vi "calibrationSpectrometer_logEvent_SummaryState.vi"(8 "error in (no error)":errorcluster, 11 "logevent_SummaryState_Ctl":T1) -> (0 "error out":errorcluster, 2 "function return":i32, 3 "logevent_SummaryState_Ctl out":T1)   [LabVIEW 2016, in "SALLV_calibrationSpectrometer.lvlib"]
doc: "int calibrationSpectrometer_shm_logEvent_SummaryStateLV(calibrationSpectrometer_logevent_SummaryStateLV *logevent_SummaryState_Ctl );"
uses:
  SALLV_calibrationSpectrometer.lvlib
  DataTypes/logevent_SummaryState.ctl
  SALLV_calibrationSpectrometer.so
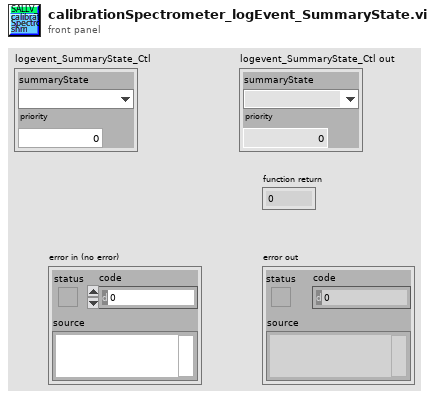
[diagram p1: front panel]
types:
  T1 = typedef "SALLV_calibrationSpectrometer.lvlib/logevent_SummaryState.ctl" = cluster{"summaryState":enum16{"", "DisabledState", "EnabledState", "FaultState", "OfflineState", "StandbyState"}, "priority":i32}
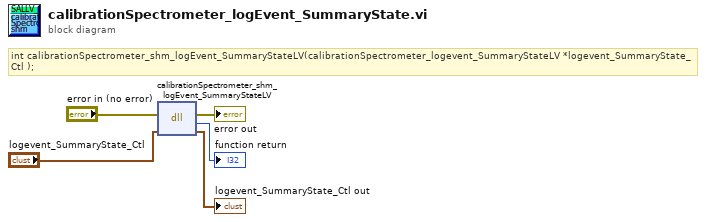
[diagram p0: block diagram]
diagram:
  # "int calibrationSpectrometer_shm_logEvent_SummaryStateLV(calibrationSpectrometer_logevent_SummaryStateLV *logevent_SummaryState_Ctl );"
  n1 = dll-call lib="home/harini/TCS/sallv_sedspectrometer/SALLV_calibrationSpectrometer.*" fn="calibrationSpectrometer_shm_logEvent_SummaryStateLV"(error in="error in (no error)", "logevent_SummaryState_Ctl"="logevent_SummaryState_Ctl") -> (error out=→"error out":errorcluster, →"function return":i32, "logevent_SummaryState_Ctl"=→"logevent_SummaryState_Ctl out":T1)  [unwired: 2 in, 1 out]
